vi "angle_enc.vi"(10 "encoder":dbl) -> (2 "angle":dbl)   [LabVIEW 2015]
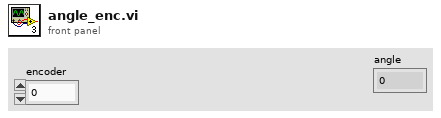
[diagram p1: front panel]
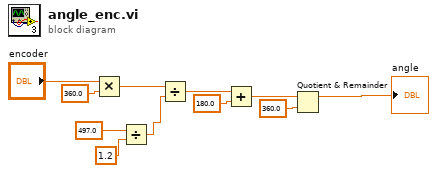
[diagram p0: block diagram]
diagram:
  n1 = Multiply(x="encoder", y=360.0) -> (x*y=w10:dbl)
  n2 = Divide(x=497.0 ("y"), y=1.2) -> (x/y=w1:dbl)
  n3 = Divide(x=w10, y=w1) -> (x/y=w8:dbl)
  n4 = Add(x=w8, y=180.0) -> (x+y=w5:dbl)
  n5 = Quotient & Remainder(x=w5, y=360.0) -> (x-y*floor(x/y)=→"angle":dbl)  [unwired: 1 out]
